vi "Created Insert.vi"(8 "Created":refnum<class "Msg Type Strategy.lvclass">, 9 "Created Alias":string, 10 "Addresses DVR in":refnum<data-value>) -> (0 "error out":errorcluster, 2 "Addresses DVR out":refnum<data-value>)   [LabVIEW 2021, in "jettl.lvlib" / "Addresses.lvlib" / "Addresses.lvclass"]
uses:
  Addresses.lvclass
  Addresses.lvclass/Addresses.ctl
  Msg Type Strategy/Msg Type Strategy/Msg Type Strategy.lvclass
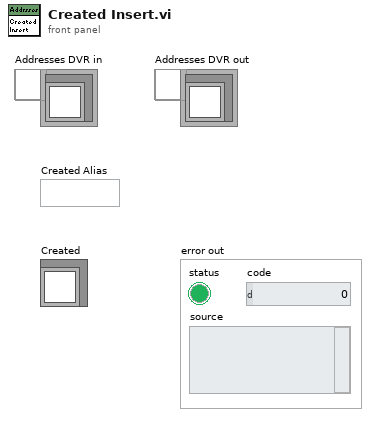
[diagram p1: front panel]
types:
  T1 = typedef "jettl.lvlib/Addresses.lvlib/Created.ctl" = map{string, refnum<class "Msg Type Strategy.lvclass">}
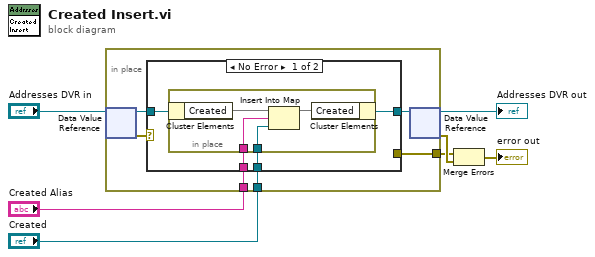
[diagram p0: block diagram]
diagram:
  n1 = in-place {
    in-place-border: [w13] -> w3
    in-place-border: "Created Alias" -> [w10]
    in-place-border: "Created" -> [w8]
    n2 = in-place-dvr #1("Addresses DVR in") -> (w11:refnum<class "Addresses.lvclass">, w12:errorcluster)
    n3 = case shown="No Error" w12 {
      selector: w12 -> [_ w23]
      tunnel: w11 -> [w15 w22]
      tunnel: [_ w23] -> w13
      tunnel: w10 -> [w17 _]
      tunnel: [w14 w22] -> w9
      tunnel: w8 -> [w16 _]
      frame No Error {
        n4 = in-place {
          in-place-border: w17 -> [w21]
          in-place-border: w16 -> [w20]
          n5 = in-place-cluster #2(w15) -> ("Created"=w19:T1)
          n6 = Insert Into Map(map in=w19, key=w21, value=w20) -> (map out=w18:T1)  [unwired: 2 out]
          n7 = in-place-cluster #2("Created"=w18) -> (w14:refnum<class "Addresses.lvclass">)
        }
      }
      frame Error {
      }
    }
    n8 = in-place-dvr #1(w9) -> (→"Addresses DVR out":refnum<data-value>, w4:errorcluster)
  }
  n9 = Merge Errors(w3, w4) -> (→"error out":errorcluster)
